vi "CH_LM Config Measurement Mode.vi"(0 "Meter Index":i32, 2 "Mode":T1, 3 "Unit":T2, 5 "error in (no error)":errorcluster, 7 "Timeout / ms (3000)":i32=1000, 8 "Action (query)":bool, 9 "Lock Timeout / ms (1000)":i32=1000) -> (11 "Lock timed out":bool, 14 "Meter Index":i32, 16 "Mode":T1, 17 "Unit":T2, 19 "error out":errorcluster)   [LabVIEW 2012, in "CH_LM.lvlib"]
doc: "This VI will query or set measurement mode and unit.\n\n<B>Attention:</B> The command will be ignored when an optical probe is attached or if a valid probe is not attached."
uses:
  CH_LM.lvlib
  CH_LM Unit.ctl
  CH_LM Measurement Mode.ctl
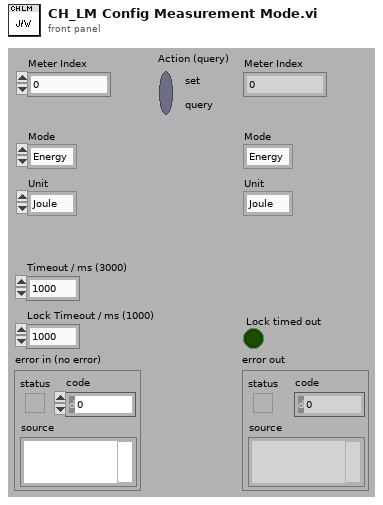
[diagram p1: front panel]
types:
  T1 = typedef "CH_LM.lvlib/CH_LM Measurement Mode.ctl" = enum16{"Energy", "Power"}
  T2 = typedef "CH_LM.lvlib/CH_LM Unit.ctl" = enum16{"Joule", "Watt", "dBm"}
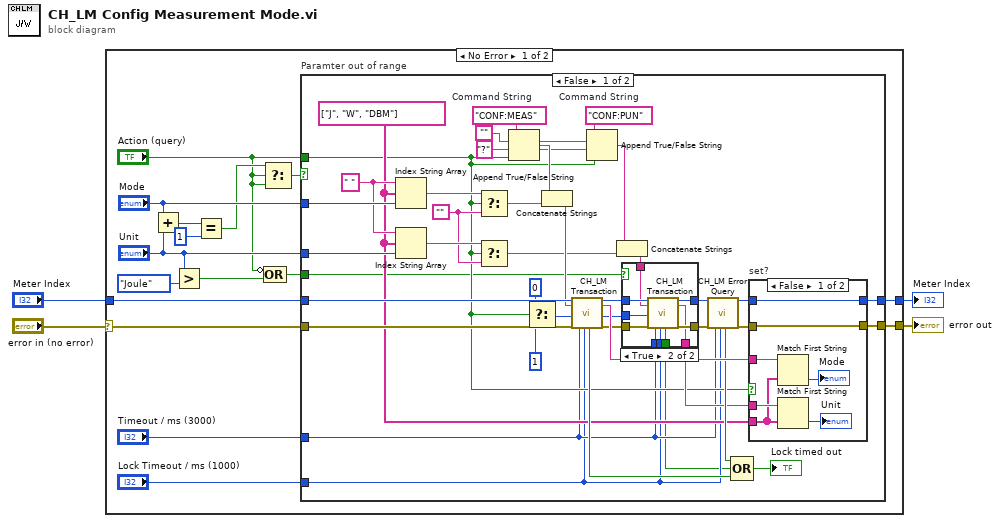
[diagram p0: block diagram]
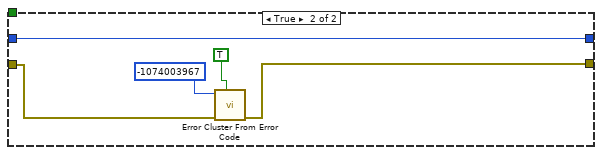
[diagram p4: hidden frame]
diagram:
  n1 = case shown="No Error" "error in (no error)" {
    selector: "error in (no error)" -> [w20 w88]
    tunnel: [w18 w88] -> w4
    tunnel: "Meter Index" -> [w19 w87]
    tunnel: [w17 w87] -> w1
    frame No Error {
      n2 = Add(x="Mode", y="Unit") -> (x+y=w12:u16)
      n3 = Greater?(x="Unit", y=CH_LM_Unit."Joule" ("Unit")) -> (0:w7:bool)
      n4 = Equal?(x=w12, y=u16 1) -> (x = y?=w11:bool)
      n5 = Select(t=w11, s="Action (query)", f="Action (query)") -> (s? t:f=w14:bool)
      n6 = Compound Arithmetic op=OR(invert "Action (query)", w7) -> (w5:bool)
      n7 = case "Paramter out of range" shown="False" w14 {
        tunnel: w20 -> [w60 w82]
        tunnel: w19 -> [w59 w86]
        tunnel: [w56 w84] -> w18
        tunnel: [w53 w86] -> w17
        tunnel: "Timeout / ms (3000)" -> [w25 _]
        tunnel: "Lock Timeout / ms (1000)" -> [w24 _]
        tunnel: "Action (query)" -> [w27 _]
        tunnel: "Mode" -> [w46 _]
        tunnel: "Unit" -> [w45 _]
        tunnel: w5 -> [w21 _]
        frame False {
          w33 = string[] ["J", "W", "DBM"]
          w30 = "CONF:PUN"  # Command String
          w34 = " " ("string (\"\")")
          w43 = ""
          w29 = ""
          w28 = "?" ("true string")
          w58 = "CONF:MEAS"  # Command String
          n8 = Index String Array(1:w46, 2:w33, 3:w34) -> (0:w47:string)
          n9 = Index String Array(1:w45, 2:w33, 3:w34) -> (0:w44:string)
          n10 = Select(t=w47, s=w27, f=w43) -> (s? t:f=w41:string)
          n11 = Select(t=w44, s=w27, f=w43) -> (s? t:f=w32:string)
          n12 = Append True/False String(1:w27, 2:w28, 3:w29, 4:w58) -> (0:w42:string)
          n13 = Select(t=0, s=w27, f=1 ("NofStrings (-1:all)")) -> (s? t:f=w22:i32)
          n14 = Concatenate Strings(w42, w41) -> (w40:string)
          n15 = call "CH_LM Transaction.vi"("Meter Index"=w59, "Command String"=w40, "NofStrings (-1:all)"=w22, "error in (no error)"=w60, "Timeout / ms (3000)"=w25, "Lock Timeout / ms (1000)"=w24) -> ("Lock timed out"=w49:bool, "Meter Index"=w39:i32, "Response"=w57:string, "error out"=w38:errorcluster)  [unwired: 10 out]
          n16 = Append True/False String(1:w27, 2:w28, 3:w29, 4:w30) -> (0:w26:string)
          n17 = Concatenate Strings(w26, w32) -> (w31:string)
          n18 = case shown="True" w21 {
            tunnel: w39 -> [w62 w72]
            tunnel: w38 -> [w61 w71]
            tunnel: [w62 w70] -> w37
            tunnel: [w61 w69] -> w36
            tunnel: [_ w68] -> w35
            tunnel: w31 -> [_ w67]
            tunnel: w25 -> [_ w66]
            tunnel: w24 -> [_ w65]
            tunnel: [_ w64] -> w23
            tunnel: w22 -> [_ w63]
            frame False {
            }
            frame True {
              n19 = call "CH_LM Transaction.vi"("Meter Index"=w72, "Command String"=w67, "NofStrings (-1:all)"=w63, "error in (no error)"=w71, "Timeout / ms (3000)"=w66, "Lock Timeout / ms (1000)"=w65) -> ("Lock timed out"=w64:bool, "Meter Index"=w70:i32, "Response"=w68:string, "error out"=w69:errorcluster)  [unwired: 10 out]
            }
          }
          n20 = call "CH_LM Error Query.vi"("Meter Index"=w37, "error in (no error)"=w36, "Timeout / ms (3000)"=w25, "Lock Timeout / ms (1000)"=w24) -> ("Lock timed out"=w50:bool, "Meter Index"=w52:i32, "error out"=w51:errorcluster)  [unwired: 13 out]
          n21 = Compound Arithmetic op=OR(w50, w23, w49) -> (→"Lock timed out":bool)
          n22 = case "set?" shown="False" w27 {
            tunnel: w57 -> [w75 _]
            tunnel: w51 -> [w78 w81]
            tunnel: [w78 w81] -> w56
            tunnel: w52 -> [w79 w80]
            tunnel: [w79 w80] -> w53
            tunnel: w35 -> [w77 _]
            tunnel: w33 -> [w73 _]
            frame False {
              n23 = Match First String(2:w73, 3:w75) -> (0:→"Mode":i32)  [unwired: 1 out]
              n24 = Match First String(2:w73, 3:w77) -> (0:→"Unit":i32)  [unwired: 1 out]
            }
            frame True {
            }
          }
        }
        frame True {
          n25 = call <vilib>:"Error Cluster From Error Code.vi"("show call chain? (False)"=TRUE, "error in (no error)"=w82, "error code (0)"=-1074003967) -> ("error out"=w84:errorcluster)  [unwired: 6 out]
        }
      }
    }
    frame Error {
    }
  }
  "error out" <- w4
  "Meter Index" <- w1
